vi "Get System Access Permission.vi"(8 "error in (no error)":errorcluster, 11 "VISA resource name":refnum<visa-resource-name>) -> (0 "error out":errorcluster, 2 "Access Permission":string, 3 "VISA resource name out":refnum<visa-resource-name>)   [LabVIEW 2020, in "Keithley 2450.lvlib"]
doc: "Returns the type of access users have to the instrument through different interfaces."
uses:
  <instrlib>/Keithley 2450/Keithley 2450.lvlib
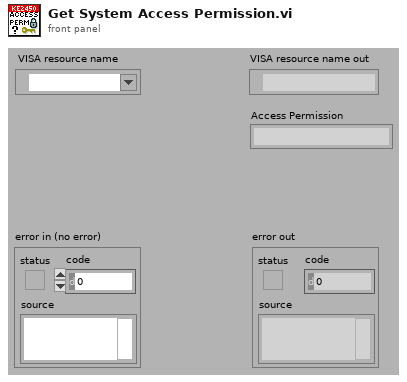
[diagram p1: front panel]
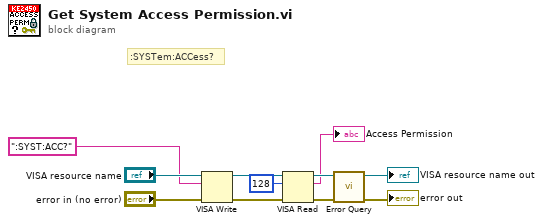
[diagram p0: block diagram]
diagram:
  # ":SYSTem:ACCess?"
  n1 = VISA Write(VISA resource name="VISA resource name", write buffer=":SYST:ACC?", error in (no error)="error in (no error)") -> (VISA resource name out=w6:refnum<visa-resource-name>, error out=w7:errorcluster)  [unwired: 1 out]
  n2 = VISA Read(VISA resource name=w6, byte count=u32 128, error in (no error)=w7) -> (VISA resource name out=w4:refnum<visa-resource-name>, read buffer=→"Access Permission":string, error out=w3:errorcluster)  [unwired: 1 out]
  n3 = call <instrlib>:"Error Query.vi"("error in (no error)"=w3, "VISA resource name"=w4) -> ("error out"=→"error out":errorcluster, "VISA resource name out"=→"VISA resource name out":refnum<visa-resource-name>)  [unwired: 8 out]
